vi "To and  From CSV.vi"() -> (0 "error out":errorcluster, 3 "Pass":bool)   [LabVIEW 2014, in "DAQmx Module Tests.lvlib"]
uses:
  DAQmx Module Tests.lvlib
  <vilib>/NI/Tag Bus Module Framework/channel/channel classification.ctl
  <vilib>/NI/Tag Bus/tag/Data Type.ctl
  <vilib>/NI/Module Execution Interface/Engine Configuration/engine configuration.lvclass
  editor node/DAQmx Module editor node.lvclass
  module/configuration/DAQmx Module Configuration.lvclass/DAQmx Module Configuration.ctl
  <vilib>/NI/Tag Bus Module Framework/channel/TBM channel.lvclass/TBM channel.ctl
  <vilib>/NI/Tag Bus/tag/tag descriptor.lvclass/tag descriptor.ctl
  <vilib>/NI/Configuration Framework/serializable configuration/NISE_CEF_serializable configuration.lvclass/NISE_CEF_serializable configuration.ctl
  <vilib>/Utility/LVClass/Get LV Class Name.vi
  <vilib>/NI/Configuration Framework/error generator/NISE_error generator.vi
  <vilib>/NI/Tag Bus Module Framework/channel/TBM channel.lvclass
  module/configuration/DAQmx Module Configuration.lvclass
  <vilib>/NI/Tag Bus/tag/tag descriptor.lvclass
  <vilib>/NI/Configuration Framework/serializable configuration/NISE_CEF_serializable configuration.lvclass
panel:
  out "data type 2":T1
  out "data type":T1
  in  "index":i32
  out "name 2":string
  out "name":string
  out "channel classification 2":T2
  out "channel classification":T2
  out "x = y?":T3(array[cluster])
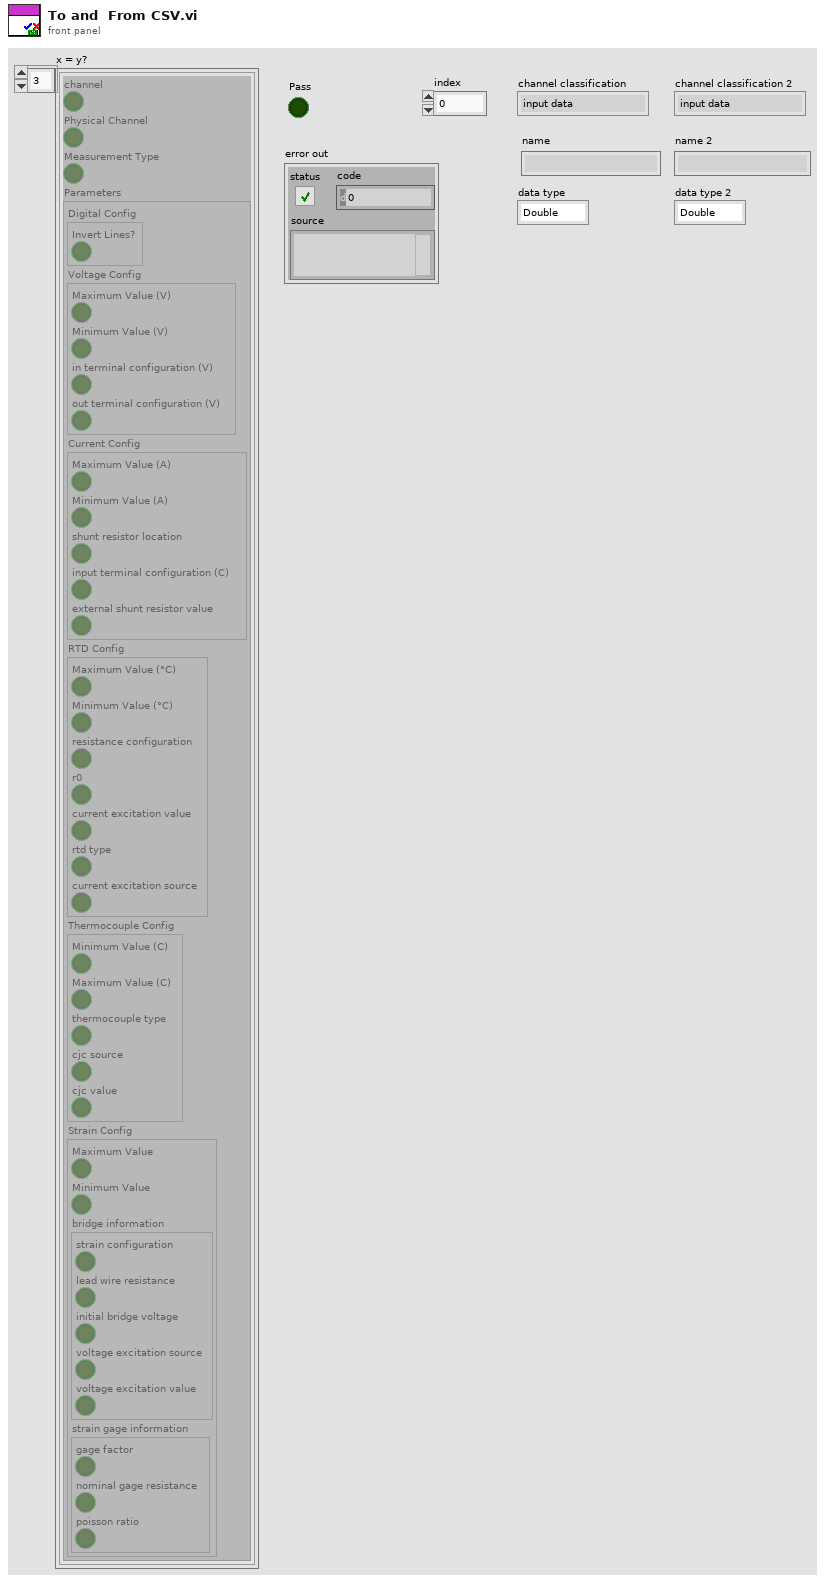
[diagram p1: front panel]
types:
  T1 = typedef "tag bus.lvlib/tag descriptor.lvclass/Data Type.ctl" = enum16{"Double", "Single", "I64", "I32", "I16", "I8", "U64", "U32", "U16", "U8", "Boolean", "String", "Array of Double", "Array of Single", "Array of I64", "Array of I32", "Array of I16", "Array of I8", "Array of U64", "Array of U32", "Array of U16", "Array of U8", "Array of Boolean", "Array of String"}
  T2 = typedef "TBM channel.lvclass/channel classification.ctl" = enum16{"input data", "output data", "processing parameter", "processing result"}
  T3 = cluster{"channel":bool, "Physical Channel":bool, "Measurement Type":bool, "Parameters":cluster{"Digital Config":cluster{"Invert Lines?":bool}, "Voltage Config":cluster{"Maximum Value (V)":bool, "Minimum Value (V)":bool, "in terminal configuration (V)":bool, "out terminal configuration (V)":bool}, "Current Config":cluster{"Maximum Value (A)":bool, "Minimum Value (A)":bool, "shunt resistor location":bool, "input terminal configuration (C)":bool, "external shunt resistor value":bool}, "RTD Config":cluster{"Maximum Value (°C)":bool, "Minimum Value (°C)":bool, "resistance configuration":bool, "r0":bool, "current excitation value":bool, "rtd type":bool, "current excitation source":bool}, "Thermocouple Config":cluster{"Minimum Value (C)":bool, "Maximum Value (C)":bool, "thermocouple type":bool, "cjc source":bool, "cjc value":bool}, "Strain Config":cluster{"Maximum Value":bool, "Minimum Value":bool, "bridge information":cluster{"strain configuration":bool, "lead wire resistance":bool, "initial bridge voltage":bool, "voltage excitation source":bool, "voltage excitation value":bool}, "strain gage information":cluster{"gage factor":bool, "nominal gage resistance":bool, "poisson ratio":bool}}}}[]
  T4 = typedef "DAQmx Module Configuration.lvclass/Line.ctl" = cluster{"channel":refnum<class "TBM channel.lvclass">, "Physical Channel":string, "Measurement Type":T5, "Parameters":T6}
  T5 = typedef "DAQmx Module Configuration.lvclass/Measurement Type.ctl" = enum16{"Digital Input", "Digital Output", "Voltage Input", "Voltage Output", "Current Input", "Current Output", "RTD", "Thermocouple", "Strain"}
  T6 = typedef "DAQmx Module Configuration.lvclass/Parameters.ctl" = cluster{"Digital Config":cluster{"Invert Lines?":bool}, "Voltage Config":cluster{"Maximum Value (V)":dbl, "Minimum Value (V)":dbl, "in terminal configuration (V)":i32, "out terminal configuration (V)":i32}, "Current Config":cluster{"Maximum Value (A)":dbl, "Minimum Value (A)":dbl, "shunt resistor location":i32, "input terminal configuration (C)":i32, "external shunt resistor value":dbl}, "RTD Config":cluster{"Maximum Value (°C)":dbl, "Minimum Value (°C)":dbl, "resistance configuration":i32, "r0":dbl, "current excitation value":dbl, "rtd type":i32, "current excitation source":i32}, "Thermocouple Config":cluster{"Minimum Value (C)":dbl, "Maximum Value (C)":dbl, "thermocouple type":i32, "cjc source":i32, "cjc value":dbl}, "Strain Config":cluster{"Maximum Value":dbl, "Minimum Value":dbl, "bridge information":cluster{"strain configuration":i32, "lead wire resistance":dbl, "initial bridge voltage":dbl, "voltage excitation source":i32, "voltage excitation value":dbl}, "strain gage information":cluster{"gage factor":dbl, "nominal gage resistance":dbl, "poisson ratio":dbl}}}
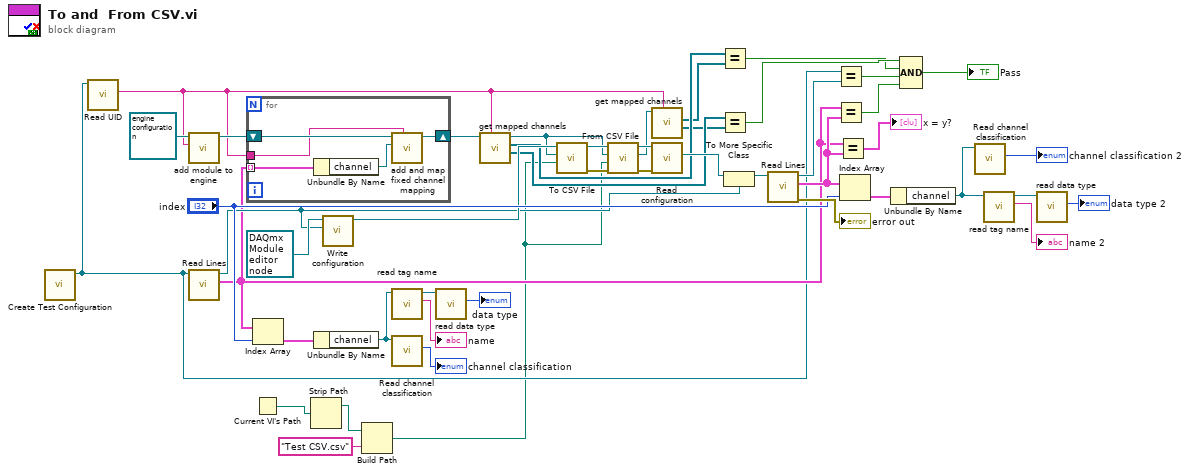
[diagram p0: block diagram]
diagram:
  n1 = call "Create Test Configuration.vi"() -> ("Module Configuration"=w15:refnum<class "DAQmx Module Configuration.lvclass">)  [unwired: 6 in, 5 out]
  n2 = call <vilib>:"Read UID.vi"("configuration in"=w15) -> ("instance id"=w9:string)  [unwired: 8 in, 2 out]
  n3 = call-dynamic "add module to engine.vi"("module ID"=w9, "engine configuration in"=refnum<class "engine configuration.lvclass"> refnum ("engine configuration")) -> ("engine configuration out"=w16:refnum<class "engine configuration.lvclass">)  [unwired: 8 in, 1 out]
  n4 = call "Read Lines.vi"("Daqmx Module configuration in"=w15) -> ("Lines"=w18:T4[], "Daqmx Module configuration out"=w19:refnum<class "DAQmx Module Configuration.lvclass">)  [unwired: 8 in, 1 out]
  n5 = for {
    tunnel: w18 -> [w52] mode=indexing
    shift-right: [w50] -> w14
    shift-left: w16 -> [w49]
    tunnel: w9 -> [w48]
    n6 = Unbundle By Name(w52) -> ("channel"=w51:refnum<class "TBM channel.lvclass">)
    n7 = call <vilib>:"add and map fixed channel mapping.vi"("module instance"=w48, "fixed channel"=w51, "engine configuration in"=w49) -> ("engine configuration out"=w50:refnum<class "engine configuration.lvclass">)  [unwired: 7 in, 1 out]
  }
  n8 = Index Array(array=w18, index="index") -> (element=w40:T4)
  n9 = Current VI's Path() -> (path=w2:path)
  n10 = Strip Path(path=w2) -> (stripped path=w1:path)  [unwired: 1 out]
  n11 = Unbundle By Name(w40) -> ("channel"=w36:refnum<class "TBM channel.lvclass">)
  n12 = call-dynamic "Write configuration.vi"("configuration"=w19, "Daqmx Module editor node in"=refnum<class "DAQmx Module editor node.lvclass"> refnum ("Daqmx Module editor node")) -> ("Daqmx Module editor node out"=w24:refnum<class "DAQmx Module editor node.lvclass">)  [unwired: 8 in, 1 out]
  n13 = Build Path(base path=w1, name or relative path="Test CSV.csv") -> (appended path=w3:path)
  n14 = call <vilib>:"read tag name.vi"("system tag in"=w36) -> ("name"=→"name":string, "system tag out"=w32:refnum<class "TBM channel.lvclass">)  [unwired: 8 in, 1 out]
  n15 = call <vilib>:"Read channel classification.vi"("channel in"=w36) -> ("channel classification"=→"channel classification":T2)  [unwired: 8 in, 2 out]
  n16 = call <vilib>:"read data type.vi"("system tag in"=w32) -> ("data type"=→"data type":T1)  [unwired: 8 in, 2 out]
  n17 = call-dynamic "get mapped channels.vi"("owner"=w9, "engine configuration in"=w14) -> ("write channels"=w8:refnum<class "TBM channel.lvclass">[], "read channels"=w11:refnum<class "TBM channel.lvclass">[], "engine configuration out"=w13:refnum<class "engine configuration.lvclass">)  [unwired: 5 in, 2 out]
  n18 = call-dynamic "To CSV File.vi"("Path"=w3, "engine configuration"=w13, "DAQmx Module Editor Node in"=w24) -> ("error out"=w27:errorcluster, "DAQmx Module Editor Node out"=w26:refnum<class "DAQmx Module editor node.lvclass">)  [unwired: 7 in]
  n19 = call-dynamic "From CSV File.vi"("error in (no error)"=w27, "Path"=w3, "engine configuration"=w13, "DAQmx Module Editor Node in"=w26) -> ("error out"=w23:errorcluster, "engine out"=w12:refnum<class "engine configuration.lvclass">, "DAQmx Module Editor Node out"=w22:refnum<class "DAQmx Module editor node.lvclass">)  [unwired: 4 in, 1 out]
  n20 = call-dynamic "get mapped channels.vi"("owner"=w9, "engine configuration in"=w12) -> ("write channels"=w7:refnum<class "TBM channel.lvclass">[], "read channels"=w10:refnum<class "TBM channel.lvclass">[])  [unwired: 5 in, 3 out]
  n21 = call-dynamic "Read configuration.vi"("error in"=w23, "Daqmx Module editor node in"=w22) -> ("configuration"=w21:refnum<class "NISE_CEF_serializable configuration.lvclass">)  [unwired: 7 in, 2 out]
  n22 = Equal?(x=w11, y=w10) -> (x = y?=w5:bool)
  n23 = Equal?(x=w8, y=w7) -> (x = y?=w6:bool)
  n24 = To More Specific Class(target class=w19, reference=w21) -> (specific class reference=w20:refnum<class "DAQmx Module Configuration.lvclass">)  [unwired: 1 in, 1 out]
  n25 = call "Read Lines.vi"("Daqmx Module configuration in"=w20) -> ("error out"=→"error out":errorcluster, "Lines"=w41:T4[], "Daqmx Module configuration out"=w46:refnum<class "DAQmx Module Configuration.lvclass">)  [unwired: 8 in]
  n26 = Equal?(x=w15, y=w46) -> (x = y?=w45:bool)
  n27 = Equal?(x=w18, y=w41) -> (x = y?=w44:bool)
  n28 = Equal?(x=w18, y=w41) -> (x = y?=→"x = y?":T3)
  n29 = Index Array(array=w41, index="index") -> (element=w39:T4)
  n30 = Unbundle By Name(w39) -> ("channel"=w35:refnum<class "TBM channel.lvclass">)
  n31 = Compound Arithmetic op=AND(w6, w5, w45, w44) -> (→"Pass":bool)
  n32 = call <vilib>:"Read channel classification.vi"("channel in"=w35) -> ("channel classification"=→"channel classification 2":T2)  [unwired: 8 in, 2 out]
  n33 = call <vilib>:"read tag name.vi"("system tag in"=w35) -> ("name"=→"name 2":string, "system tag out"=w31:refnum<class "TBM channel.lvclass">)  [unwired: 8 in, 1 out]
  n34 = call <vilib>:"read data type.vi"("system tag in"=w31) -> ("data type"=→"data type 2":T1)  [unwired: 8 in, 2 out]
